vi "Test_State_Block_Chain.vi"() -> ()   [LabVIEW 2021]
uses:
  C:/Program Files (x86)/Hyper State Machine Framework/SSW_Hyper_State_Machine.lvlibp/State_Machine_Class/Main_State_Machine/Hyper_State_Machine.lvclass
  C:/Program Files (x86)/Hyper State Machine Framework/SSW_Hyper_State_Machine.lvlibp/State_Interface/State_Interface.lvclass
  Motion_Panel_State_Machine/Motion_Panel_State_Machine.lvclass
  C:/Program Files (x86)/Hyper State Machine Framework/SSW_Panel_Adaptive.lvlibp/Panel_Adaptive/Panel_Adaptive.lvclass
  C:/Program Files (x86)/Hyper State Machine Framework/SSW_Panel_Adaptive.lvlibp/Panel_Interface/Panel_Interface.lvclass
  DIO_Panel_State_Machine/DIO_Panel_State_Machine.lvclass
  Class 1/Panel1.lvclass
  Class 3/Panel3.lvclass
  Class 2/Panel2.lvclass
  C:/Program Files (x86)/Hyper State Machine Framework/SSW_Hyper_State_Machine.lvlibp/State_Machine_Class/State_Machine_Module.llb/State Machine.ctl
  C:/Program Files (x86)/Hyper State Machine Framework/SSW_Hyper_State_Machine.lvlibp/State_Machine_Class/State_Machine_Module.llb/State Machine[].ctl
  C:/Program Files (x86)/Hyper State Machine Framework/SSW_Hyper_State_Machine.lvlibp/State_Machine_Class/State_Machine_Module.llb/Time_Out.ctl
  C:/Program Files (x86)/Hyper State Machine Framework/SSW_Hyper_State_Machine.lvlibp/State_Machine_Class/State_Machine_Module.llb/Lock_Unlock.ctl
  C:/Program Files (x86)/Hyper State Machine Framework/SSW_Hyper_State_Machine.lvlibp
panel:
  out "Parent_State":refnum<class "Hyper_State_Machine.lvclass">
  out "HPSMO4-20":refnum<class "Panel_Adaptive.lvclass">[](array[class])
  out "HPSMO2":refnum<class "Panel_Adaptive.lvclass">
  out "HSMO4-20":refnum<class "Hyper_State_Machine.lvclass">[](array[class])
  out "HSMO3":refnum<class "Hyper_State_Machine.lvclass">
  out "HPSMO3":refnum<class "DIO_Panel_State_Machine.lvclass">
  out "HSMO2":refnum<class "Hyper_State_Machine.lvclass">
  out "HSMO1":refnum<class "Hyper_State_Machine.lvclass">
  out "HPSMO1":refnum<class "Motion_Panel_State_Machine.lvclass">
  in  "Reset_State":bool
  in  "Reset_All":bool
  in  "Change_VI_All":bool
  in  "Panel Index":i32=1 min=1 max=20
  in  "Implementation":u16(ring)
  in  "Change_VI":bool
  out "Main_Active":bool
  in  "Main_Interval(s)":dbl=0.025 format="%.0p"
  in  "Option Button":bool=TRUE
  in  "Time Target (s)":dbl=30.0 format="%#_13g"
  in  "lock All":bool
  in  "Unlock":bool
  out "All_Values":variant[][](array[variant])
  out "error out":errorcluster
  in  "Exit":bool
  in  "Tab Control":T1(tab)
  in  "Panel Mode 4":bool
  in  "Panel Mode 3":bool
  in  "Panel Mode 2":bool
  in  "Panel Mode 1":bool
  in  "Swap3-4":bool
  in  "Swap1-4":bool
  in  "Swap2-3":bool
  in  "Swap1-2":bool
  out "Active 3":bool
  out "Active 2":bool
  out "Timing 3":dbl
  out "Timing 2":dbl
  out "Active 1":bool
  out "Timing 1":dbl
  out "Timing 20":dbl
  out "Active 20":bool
  out "Get_Current State_Sub Panel_1":string
  out "Sub Panel_1(HSMO_ID)":u32 format="%08x"
  out "HSMO1 Running":bool
  in  "Request_Release(Index)":bool
  out "Block_Chain_Lock":bool
  out "Current_Parent_State":string
  out "Parent_State_ID":u32 format="%08x"
  out "Received State Message":string
  out "Child_State#":u32
  out "Child_State_ID":u32[](array[numeric]) format="%.0x"
  in  "Panel_Index":u32 max=3 step=1
  # "Local"
  # "Panel Method"
  # "State Method"
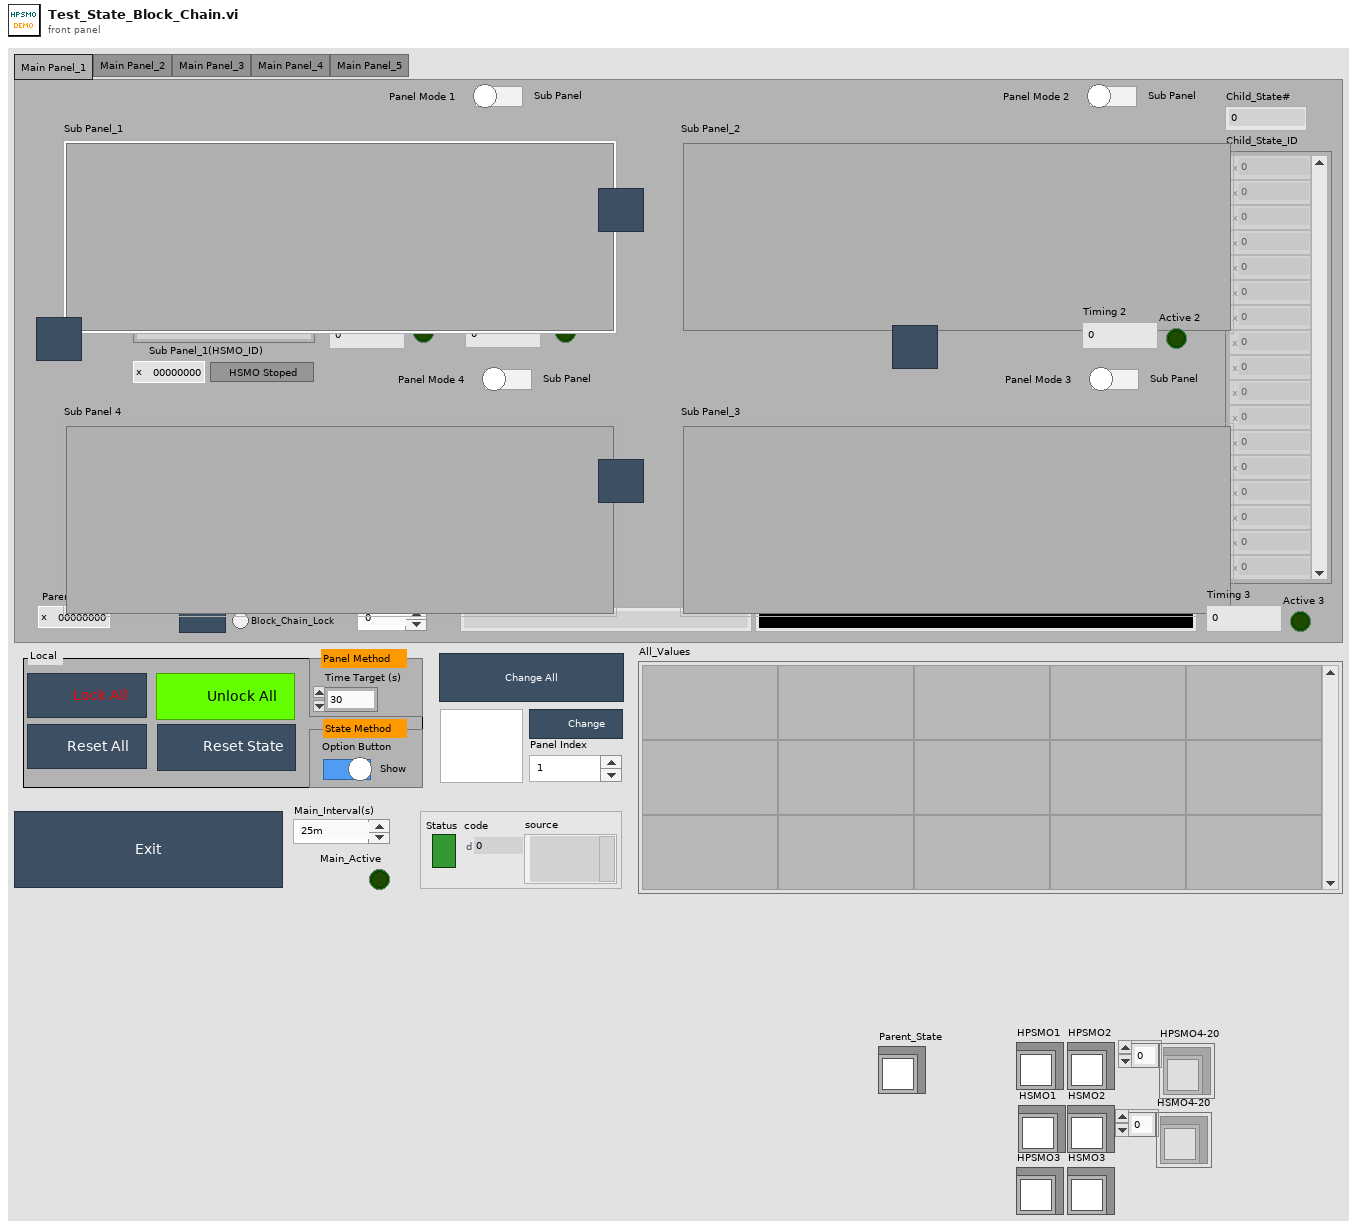
[diagram p1: front panel]
types:
  T1 = enum32{"Main Panel_1", "Main Panel_2", "Main Panel_3", "Main Panel_4", "Main Panel_5"}
  T2 = typedef "SSW_Hyper_State_Machine.lvlibp/State Machine.ctl" = cluster{"Command":string, "Data":variant}
  T3 = typedef "SSW_Hyper_State_Machine.lvlibp/Lock_Unlock.ctl" = cluster{"Action_Mode (Get)":enum16{"Set", "Get"}, "Action_Set (False)":bool, "State_In (Wait)":string}
  T4 = typedef "SSW_Hyper_State_Machine.lvlibp/State Machine[].ctl" = cluster{"Command":string, "Data":variant}[]
  T5 = typedef "SSW_Hyper_State_Machine.lvlibp/Time_Out.ctl" = cluster{"Enable(True)":bool, "Time Out_State Name":string, "Time Target (1s)":dbl, "Time Out_Reply Message_State":string}
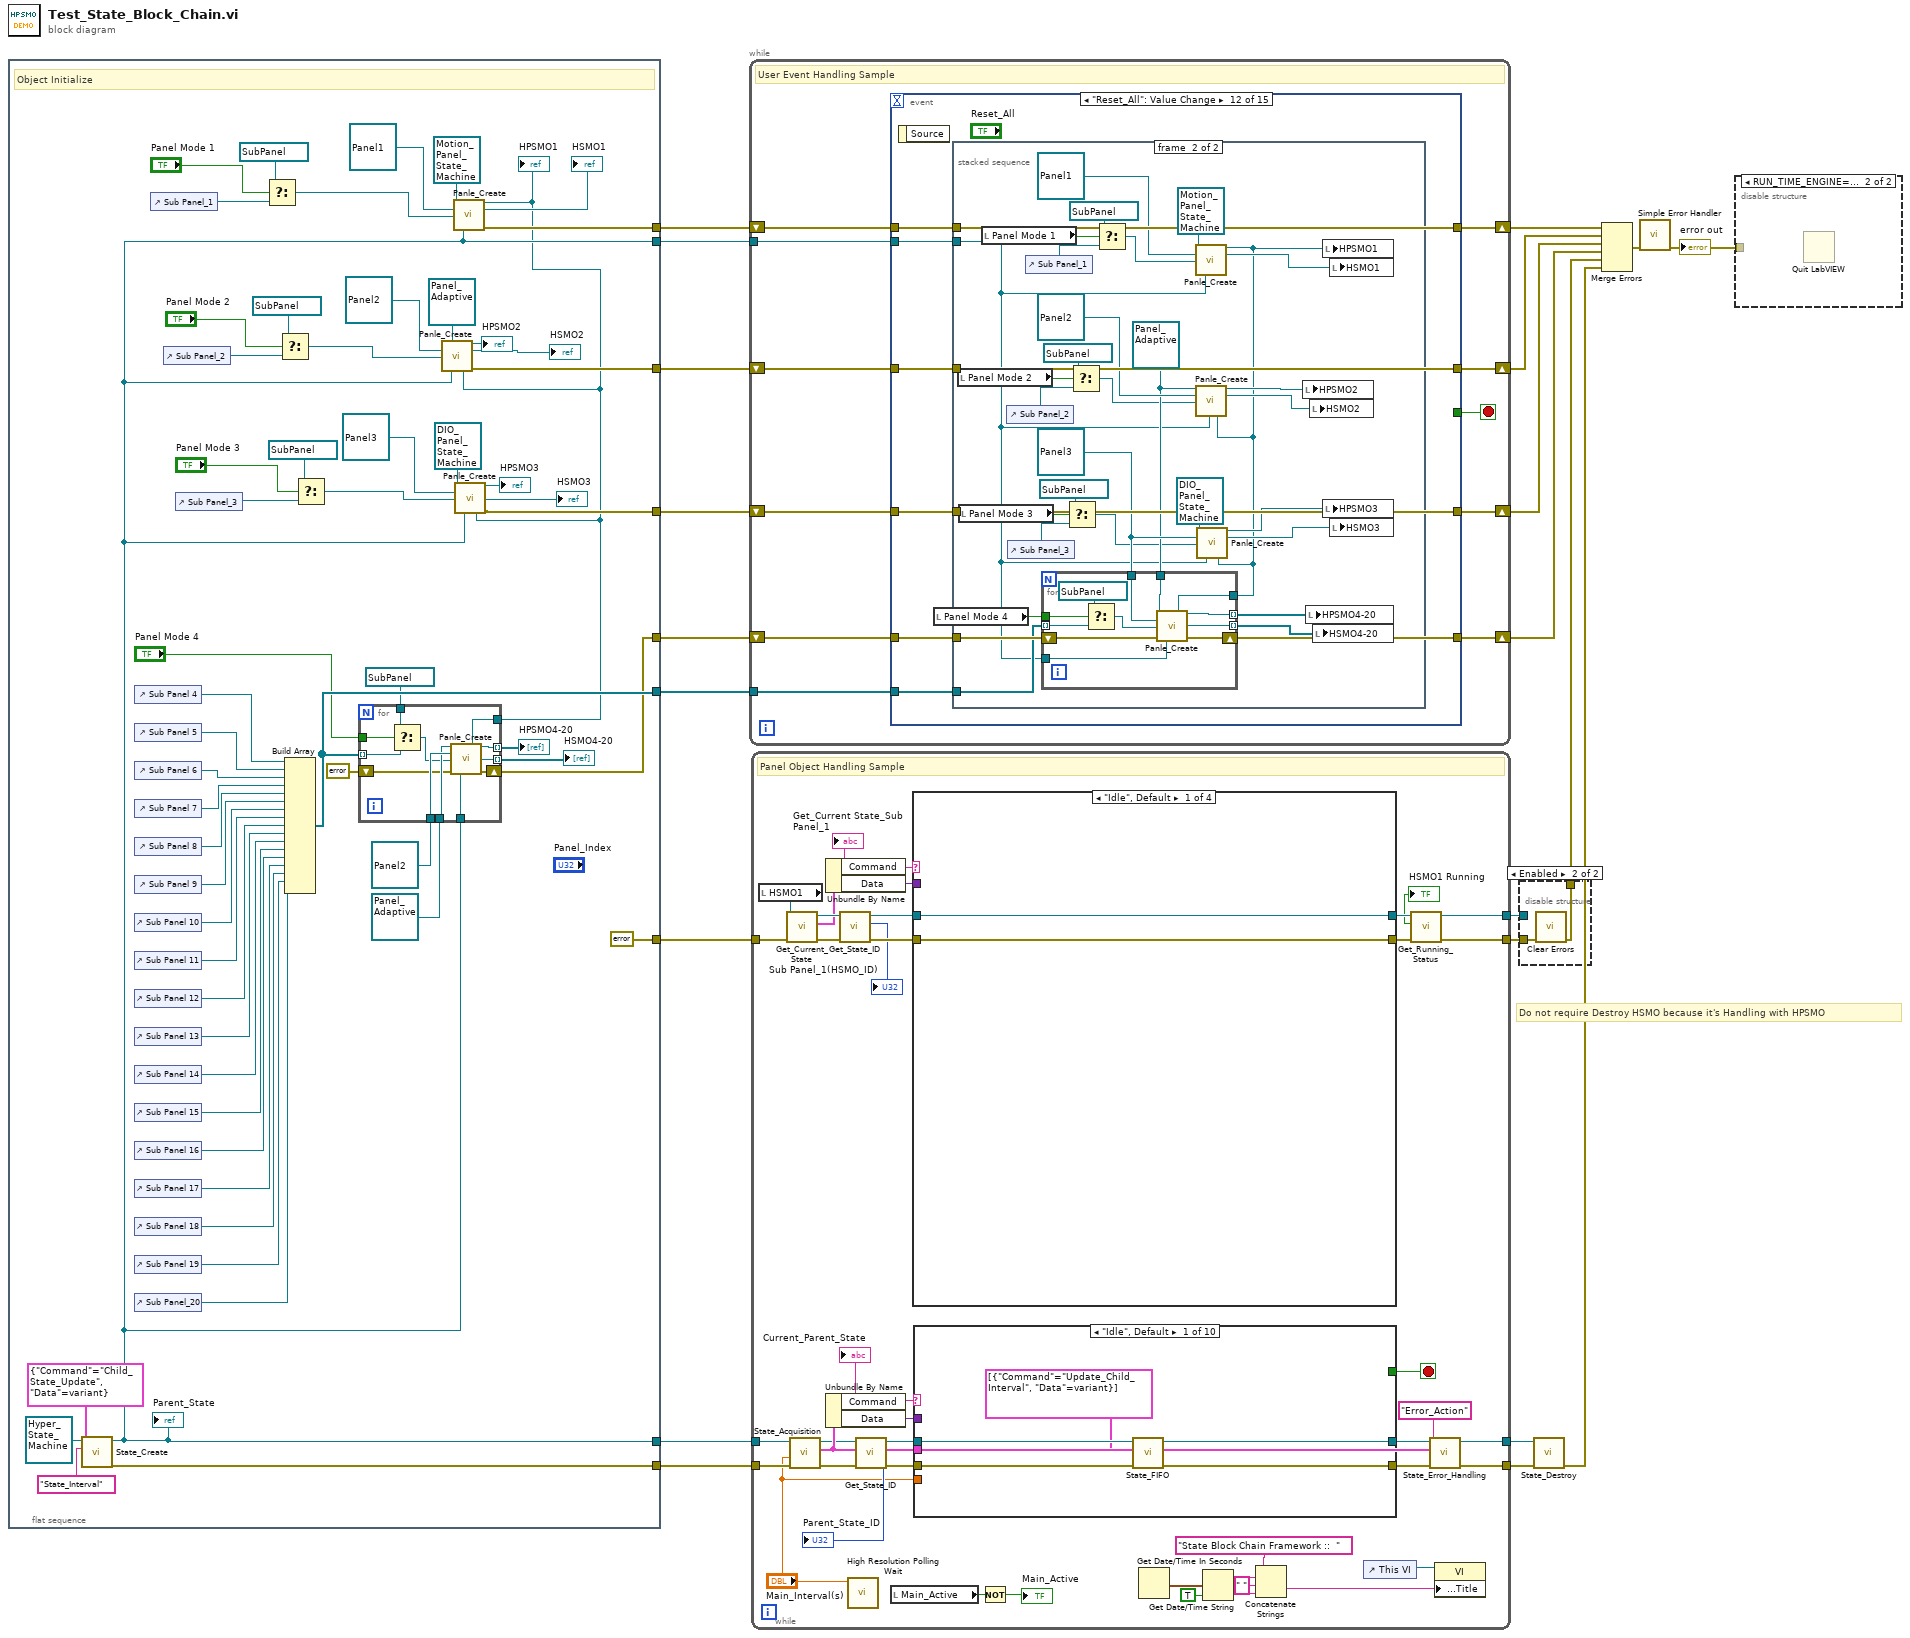
[diagram p0: block diagram]
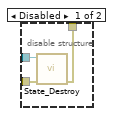
[diagram p2: hidden frame]
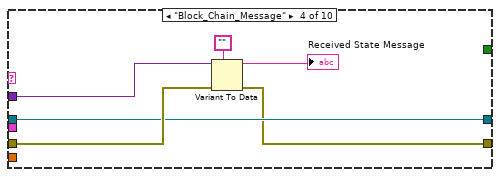
[diagram p6: hidden frame]
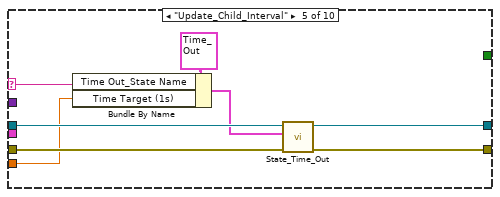
[diagram p7: hidden frame]
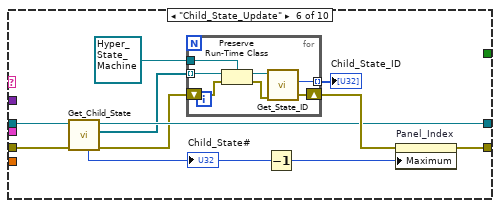
[diagram p8: hidden frame]
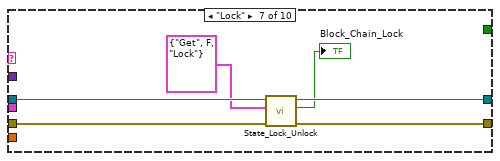
[diagram p9: hidden frame]
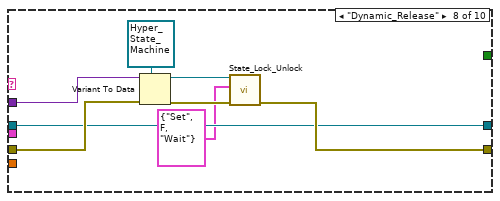
[diagram p10: hidden frame]
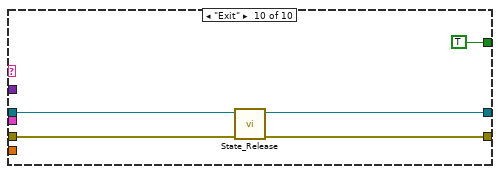
[diagram p12: hidden frame]
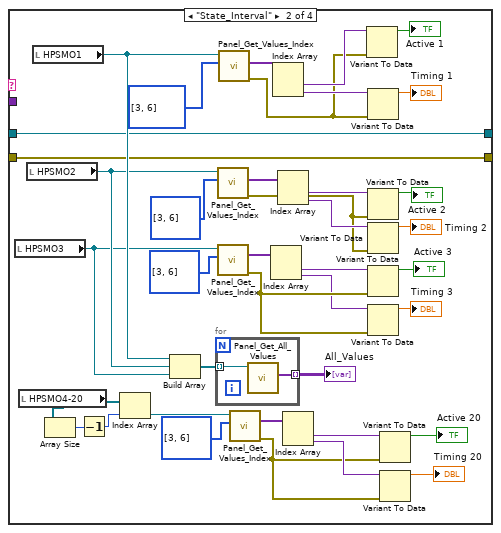
[diagram p13: hidden frame]
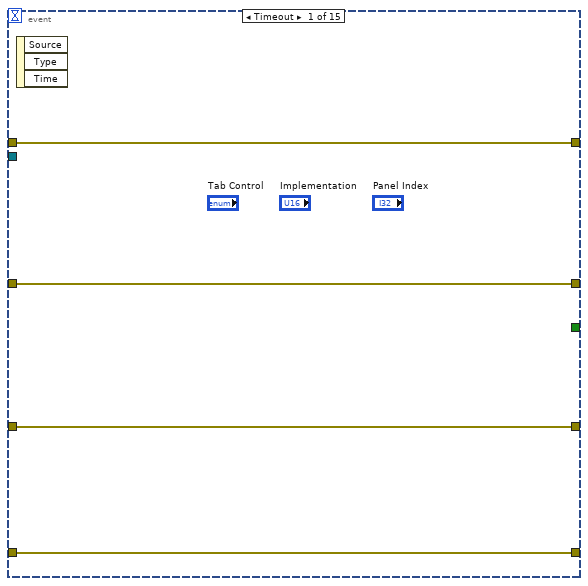
[diagram p16: hidden frame]
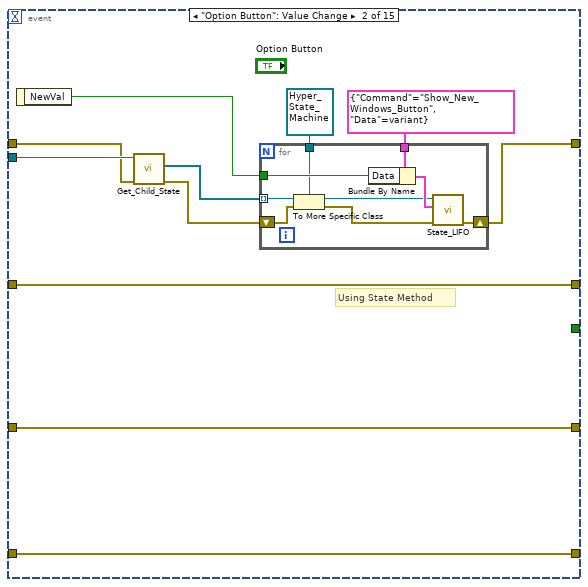
[diagram p17: hidden frame]
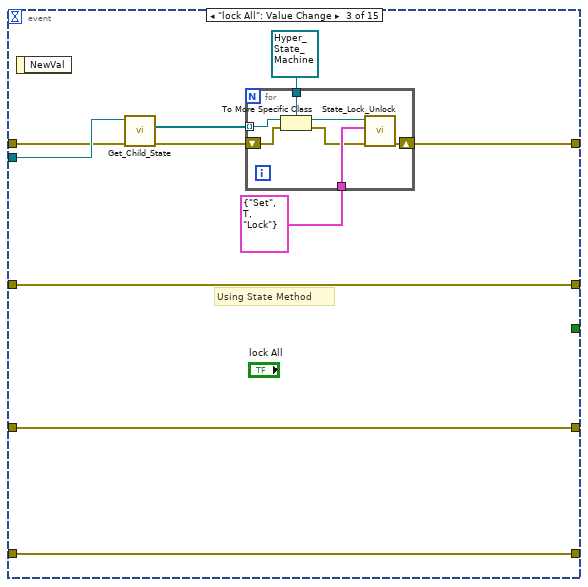
[diagram p18: hidden frame]
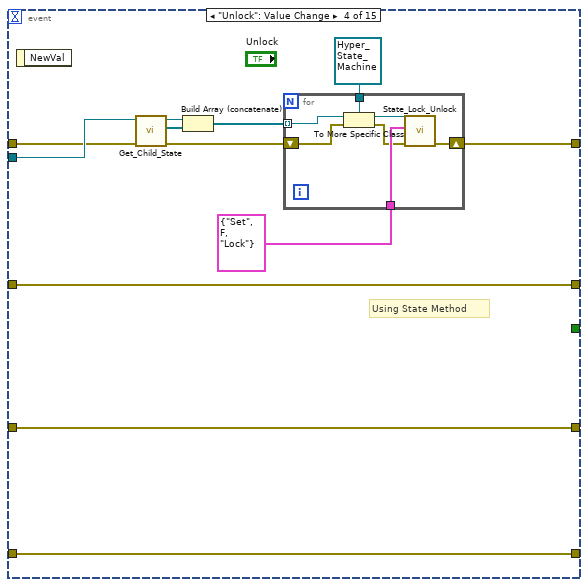
[diagram p19: hidden frame]
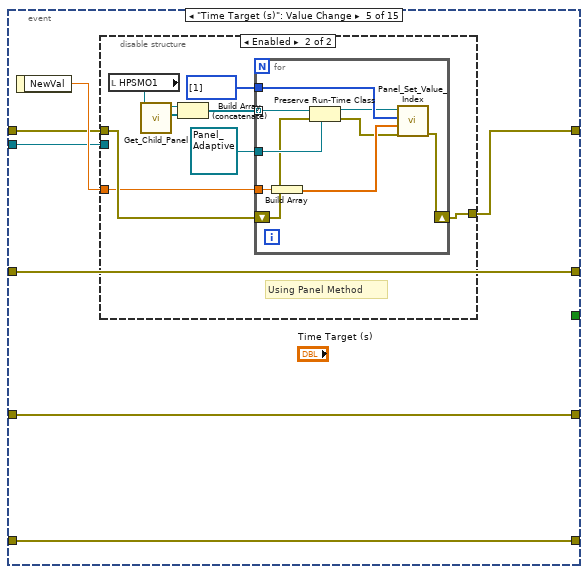
[diagram p20: hidden frame]
diagram:
  # "Do not require Destroy HSMO because it's Handling with HPSMO"
  n1 = flat-sequence {
    tunnel: [w55] -> w21
    tunnel: [w53] -> w10
    tunnel: [w52] -> w7
    tunnel: [w51] -> w8
    tunnel: [w46] -> w9
    tunnel: [errorcluster {"status"=FALSE, "code"=0, "source"=""} ("error in (no error)")] -> w14
    tunnel: [w37] -> w13
    tunnel: [w39] -> w12
    tunnel: [w37] -> w11
    frame #0 {
      # "Object Initialize"
      n2 = call-dynamic "State_Create.vi"("Init_State(Option)"=T2 {"Command"="Child_State_Update", "Data"=variant}, "State_Interval_Name"="State_Interval", "State_Machine_Class in"=refnum<class "Hyper_State_Machine.lvclass"> refnum) -> ("error out"=w39:errorcluster, "State_Machine_Class out"=w37:refnum<class "Hyper_State_Machine.lvclass">)  [unwired: 6 in, 1 out]
      "Parent_State" <- w37
      n3 = control-ref of="Sub Panel 4"() -> (w75:refnum<vi>)
      n4 = control-ref of="Sub Panel 5"() -> (w74:refnum<vi>)
      n5 = control-ref of="Sub Panel 6"() -> (w73:refnum<vi>)
      n6 = control-ref of="Sub Panel 7"() -> (w72:refnum<vi>)
      n7 = control-ref of="Sub Panel 8"() -> (w71:refnum<vi>)
      n8 = control-ref of="Sub Panel 9"() -> (w70:refnum<vi>)
      n9 = control-ref of="Sub Panel 10"() -> (w69:refnum<vi>)
      n10 = control-ref of="Sub Panel 11"() -> (w68:refnum<vi>)
      n11 = control-ref of="Sub Panel 12"() -> (w67:refnum<vi>)
      n12 = control-ref of="Sub Panel 13"() -> (w66:refnum<vi>)
      n13 = control-ref of="Sub Panel 14"() -> (w65:refnum<vi>)
      n14 = control-ref of="Sub Panel 15"() -> (w64:refnum<vi>)
      n15 = control-ref of="Sub Panel 16"() -> (w63:refnum<vi>)
      n16 = control-ref of="Sub Panel 17"() -> (w62:refnum<vi>)
      n17 = control-ref of="Sub Panel 18"() -> (w61:refnum<vi>)
      n18 = control-ref of="Sub Panel 19"() -> (w60:refnum<vi>)
      n19 = control-ref of="Sub Panel_20"() -> (w58:refnum<vi>)
      n20 = control-ref of="Sub Panel_1"() -> (w35:refnum<vi>)
      n21 = control-ref of="Sub Panel_2"() -> (w30:refnum<vi>)
      n22 = control-ref of="Sub Panel_3"() -> (w26:refnum<vi>)
      n23 = Select(t=refnum<vi> refnum, s="Panel Mode 1", f=w35) -> (s? t:f=w34:refnum<vi>)
      n24 = Select(t=refnum<vi> refnum, s="Panel Mode 2", f=w30) -> (s? t:f=w28:refnum<vi>)
      n25 = Build Array(w75, w74, w73, w72, w71, w70, w69, w68, w67, w66, w65, w64, w63, w62, w61, w60, w58) -> (w55:refnum<vi>[])
      n26 = Select(t=refnum<vi> refnum, s="Panel Mode 3", f=w26) -> (s? t:f=w25:refnum<vi>)
      n27 = call-dynamic "Panle_Create.vi"("Hyper_Panel_State_Machine in"=refnum<class "Motion_Panel_State_Machine.lvclass"> refnum ("Motion_Panel_State_Machine.lvclass"), "Panel_Source"=refnum<class "Panel1.lvclass"> refnum ("Class 1.lvclass"), "Panel_Ref"=w34, "Parent_State"=w37) -> ("Hyper_Panel_State_Machine out"=w22:refnum<class "Motion_Panel_State_Machine.lvclass">, "This_State"=→"HSMO1":refnum<class "Hyper_State_Machine.lvclass">, "error out"=w53:errorcluster)  [unwired: 9 in]
      "HPSMO1" <- w22
      n28 = for {
        shift-right: [w89] -> w52
        shift-left: errorcluster {"status"=FALSE, "code"=0, "source"=""} ("error out") -> [w90]
        tunnel: w55 -> [w84] mode=indexing
        tunnel: [w88] -> w59 mode=indexing
        tunnel: refnum<class "Panel2.lvclass"> refnum ("Class 2.lvclass") -> [w92]
        tunnel: refnum<class "Panel_Adaptive.lvclass"> refnum ("SSW_Panel_Adaptive.lvlibp:Panel_Adaptive.lvclass") -> [w91]
        tunnel: [w87] -> w44 mode=indexing
        tunnel: w37 -> [w86]
        tunnel: "Panel Mode 4" -> [w85]
        tunnel: refnum<vi> refnum ("t") -> [w83]
        tunnel: w22 -> [w81]
        n29 = Select(t=w83, s=w85, f=w84) -> (s? t:f=w82:refnum<vi>)
        n30 = call-dynamic "Panle_Create.vi"("Hyper_Panel_State_Machine in"=w91, "Panel_Source"=w92, "Panel_Ref"=w82, "error in (no error)"=w90, "Parent_State"=w86, "Parent_Panel"=w81) -> ("Hyper_Panel_State_Machine out"=w87:refnum<class "Panel_Adaptive.lvclass">, "This_State"=w88:refnum<class "Hyper_State_Machine.lvclass">, "error out"=w89:errorcluster)  [unwired: 7 in]
      }
      "HSMO4-20" <- w59
      "HPSMO4-20" <- w44
      n31 = call-dynamic "Panle_Create.vi"("Hyper_Panel_State_Machine in"=refnum<class "Panel_Adaptive.lvclass"> refnum ("SSW_Panel_Adaptive.lvlibp:Panel_Adaptive.lvclass"), "Panel_Source"=refnum<class "Panel2.lvclass"> refnum ("Class 2.lvclass"), "Panel_Ref"=w28, "Parent_State"=w37, "Parent_Panel"=w22) -> ("Hyper_Panel_State_Machine out"=→"HPSMO2":refnum<class "Panel_Adaptive.lvclass">, "This_State"=→"HSMO2":refnum<class "Hyper_State_Machine.lvclass">, "error out"=w46:errorcluster)  [unwired: 8 in]
      n32 = call-dynamic "Panle_Create.vi"("Hyper_Panel_State_Machine in"=refnum<class "DIO_Panel_State_Machine.lvclass"> refnum ("DIO_Panel_State_Machine.lvclass"), "Panel_Source"=refnum<class "Panel3.lvclass"> refnum ("Class 3.lvclass"), "Panel_Ref"=w25, "Parent_State"=w37, "Parent_Panel"=w22) -> ("Hyper_Panel_State_Machine out"=→"HPSMO3":refnum<class "DIO_Panel_State_Machine.lvclass">, "This_State"=→"HSMO3":refnum<class "Hyper_State_Machine.lvclass">, "error out"=w51:errorcluster)  [unwired: 8 in]
    }
  }
  n33 = while {
    tunnel: w21 -> [w102]
    tunnel: w11 -> [w101]
    shift-right: [w93] -> w3
    shift-left: w10 -> [w100]
    shift-right: [w94] -> w4
    shift-left: w9 -> [w99]
    shift-right: [w95] -> w5
    shift-left: w8 -> [w98]
    shift-right: [w96] -> w6
    shift-left: w7 -> [w97]
    stop <- w103 stop-if-true
    # "User Event Handling Sample"
    n34 = event shown="[11] \"Reset_All\": Value Change" {
      selector: _ -> [_ _ _ _ _ _ _ _ _ _ _ _ _ _ _]
      dyn-events: _ -> [_ _ _ _ _ _ _ _ _ _ _ _ _ _ _]
      timeout: _ -> [_ _ _ _ _ _ _ _ _ _ _ _ _ _ _]
      tunnel: [_ _ _ _ _ _ _ _ _ _ _ _ _ _ w384] -> w103
      tunnel: w100 -> [w105 w110 w130 w148 w168 w213 _ w252 w257 w273 w281 w290 w348 w376 w392]
      tunnel: [_ w118 w137 w156 w170 w219 w232 w251 w257 w270 w281 w290 w351 w380 w390] -> w93
      tunnel: w99 -> [w106 w115 w135 w154 w165 _ _ w247 w262 w268 w282 w289 w355 _ w387]
      tunnel: [w105 _ _ _ _ _ _ _ _ _ _ _ _ _ _] -> _
      tunnel: [w106 w115 w135 w154 w165 w219 w232 w250 w260 w268 w282 w289 w355 _ w389] -> w94
      tunnel: [w107 w114 w134 w153 w166 w219 w232 w249 w259 w269 w280 w288 w354 _ w388] -> w95
      tunnel: w97 -> [w104 w113 w133 w152 w167 _ _ w248 w258 w272 w284 w287 w353 _ w386]
      tunnel: [w104 w113 w133 w152 w167 w219 w232 w248 w258 w271 w283 w287 w353 _ w385] -> w96
      tunnel: w98 -> [w107 w114 w134 w153 w166 _ _ w249 w261 w269 w279 w288 w354 _ w391]
      tunnel: w102 -> [_ _ _ _ _ _ _ _ _ _ _ w286 _ _ _]
      tunnel: w101 -> [_ w111 w131 w149 w164 _ _ _ _ _ _ w285 w349 w377 w382]
      event Timeout {
        n35 = event-data() -> ()  [unwired: 1 in, 3 out]
      }
      event "Option Button": Value Change {
        # "Using State Method"
        n36 = event-data() -> ("NewVal"=w117:bool)  [unwired: 1 in]
        n37 = call-dynamic "Get_Child_State.vi"("error in (no error)"=w110, "Hyper_State_Machine in"=w111) -> ("error out"=w108:errorcluster, "Child_State"=w109:refnum<class "State_Interface.lvclass">[])  [unwired: 5 in, 3 out]
        n38 = for {
          tunnel: w117 -> [w126]
          tunnel: w109 -> [w123] mode=indexing
          shift-right: [w127] -> w118
          shift-left: w108 -> [w120]
          tunnel: T2 {"Command"="Show_New_Windows_Button", "Data"=variant} ("State Machine") -> [w124]
          tunnel: refnum<class "Hyper_State_Machine.lvclass"> refnum ("HSMO1") -> [w122]
          n39 = To More Specific Class(target class=w122, reference=w123, error in=w120) -> (specific class reference=w121:refnum<class "Hyper_State_Machine.lvclass">, error out=w119:errorcluster)
          n40 = Bundle By Name(cluster=w124, "Data"=w126) -> (w125:T2)
          n41 = call-dynamic "State_LIFO.vi"("error in (no error)"=w119, "State Machine"=w125, "State_Machine_Class in"=w121) -> ("error out"=w127:errorcluster)  [unwired: 7 in, 1 out]
        }
      }
      event "lock All": Value Change {
        # "Using State Method"
        n42 = event-data() -> ()  [unwired: 1 in, 1 out]
        n43 = call-dynamic "Get_Child_State.vi"("error in (no error)"=w130, "Hyper_State_Machine in"=w131) -> ("error out"=w128:errorcluster, "Child_State"=w129:refnum<class "State_Interface.lvclass">[])  [unwired: 5 in, 3 out]
        n44 = for {
          shift-right: [w144] -> w137
          shift-left: w128 -> [w139]
          tunnel: T3 {"Action_Mode (Get)"=enum."Set", "Action_Set (False)"=TRUE, "State_In (Wait)"="Lock"} ("Parameter") -> [w143]
          tunnel: refnum<class "Hyper_State_Machine.lvclass"> refnum ("HSMO1") -> [w142]
          tunnel: w129 -> [w140] mode=indexing
          n45 = To More Specific Class(target class=w142, reference=w140, error in=w139) -> (specific class reference=w141:refnum<class "Hyper_State_Machine.lvclass">, error out=w138:errorcluster)
          n46 = call-dynamic "State_Lock_Unlock.vi"("error in (no error)"=w138, "Parameter"=w143, "State_Machine_Class in"=w141) -> ("error out"=w144:errorcluster)  [unwired: 6 in, 2 out]
        }
      }
      event "Unlock": Value Change {
        # "Using State Method"
        n47 = event-data() -> ()  [unwired: 1 in, 1 out]
        n48 = call-dynamic "Get_Child_State.vi"("error in (no error)"=w148, "Hyper_State_Machine in"=w149) -> ("error out"=w147:errorcluster, "Child_State"=w145:refnum<class "State_Interface.lvclass">[], "Hyper_State_Machine out"=w146:refnum<class "Hyper_State_Machine.lvclass">)  [unwired: 5 in, 2 out]
        n49 = Build Array (concatenate)(w146, w145) -> (w150:refnum<class "State_Interface.lvclass">[])
        n50 = for {
          shift-right: [w163] -> w156
          shift-left: w147 -> [w158]
          tunnel: T3 {"Action_Mode (Get)"=enum."Set", "Action_Set (False)"=FALSE, "State_In (Wait)"="Lock"} ("Parameter") -> [w162]
          tunnel: refnum<class "Hyper_State_Machine.lvclass"> refnum ("HSMO1") -> [w161]
          tunnel: w150 -> [w157] mode=indexing
          n51 = To More Specific Class(target class=w161, reference=w157, error in=w158) -> (specific class reference=w160:refnum<class "Hyper_State_Machine.lvclass">, error out=w159:errorcluster)
          n52 = call-dynamic "State_Lock_Unlock.vi"("error in (no error)"=w159, "Parameter"=w162, "State_Machine_Class in"=w160) -> ("error out"=w163:errorcluster)  [unwired: 6 in, 2 out]
        }
      }
      event "Time Target (s)": Value Change {
        n53 = event-data() -> ("NewVal"=w169:dbl)  [unwired: 1 in]
        n54 = disable-structure shown="Enabled" {
          disable-tunnel: [w177 w194] -> w170
          disable-tunnel: w169 -> [w178 w195]
          disable-tunnel: w168 -> [w173 w196]
          disable-tunnel: w164 -> [w174 _]
          frame Disabled {
            # "Using State Method"
            n55 = call-dynamic "Get_Child_State.vi"("error in (no error)"=w173, "Hyper_State_Machine in"=w174) -> ("error out"=w172:errorcluster, "Child_State"=w171:refnum<class "State_Interface.lvclass">[])  [unwired: 5 in, 3 out]
            n56 = for {
              tunnel: w178 -> [w187]
              shift-right: [w186] -> w177
              shift-left: w172 -> [w180]
              tunnel: T2 {"Command"="Change_Time_Target", "Data"=variant} ("State Machine") -> [w184]
              tunnel: w171 -> [w183] mode=indexing
              tunnel: refnum<class "Hyper_State_Machine.lvclass"> refnum ("HSMO1") -> [w181]
              n57 = To More Specific Class(target class=w181, reference=w183, error in=w180) -> (specific class reference=w182:refnum<class "Hyper_State_Machine.lvclass">, error out=w179:errorcluster)
              n58 = Bundle By Name(cluster=w184, "Data"=w187) -> (w185:T2)
              n59 = call-dynamic "State_LIFO.vi"("error in (no error)"=w179, "State Machine"=w185, "State_Machine_Class in"=w182) -> ("error out"=w186:errorcluster)  [unwired: 7 in, 1 out]
            }
          }
          frame Enabled {
            # "Using Panel Method"
            n60 = local read "HPSMO1"() -> (w188:refnum<class "Motion_Panel_State_Machine.lvclass">)
            n61 = call-dynamic "Get_Child_Panel.vi"("Motion_Panel_State_Machine in"=w188) -> ("Child_Panel"=w192:refnum<class "Panel_Interface.lvclass">[], "Motion_Panel_State_Machine out"=w191:refnum<class "Motion_Panel_State_Machine.lvclass">)  [unwired: 6 in, 3 out]
            n62 = Build Array (concatenate)(w191, w192) -> (w190:refnum<class "Panel_Interface.lvclass">[])
            n63 = for {
              tunnel: w190 -> [w201] mode=indexing
              tunnel: w195 -> [w205]
              shift-right: [w202] -> w194
              shift-left: w196 -> [w199]
              tunnel: i32[] [1] ("Control_Indexes(Tabbing Order)") -> [w204]
              tunnel: refnum<class "Panel_Adaptive.lvclass"> refnum ("SSW_Panel_Adaptive.lvlibp:Panel_Adaptive.lvclass") -> [w200]
              n64 = Build Array(w205) -> (w203:dbl[])
              n65 = Preserve Run-Time Class(object in=w201, error in=w199, 2:w200) -> (object out=w198:refnum<class "Panel_Adaptive.lvclass">, error out=w197:errorcluster)
              n66 = call-dynamic "Panel_Set_Value_Index.vi"("error in (no error)"=w197, "Data_Values"=w203, "Control_Indexes(Tabbing Order)"=w204, "Hyper_Panel_State_Machine in"=w198) -> ("error out"=w202:errorcluster)  [unwired: 6 in, 1 out]
            }
          }
        }
      }
      event "Change_VI": Value Change {
        n67 = event-data() -> ()  [unwired: 1 in, 1 out]
        n68 = local read "Implementation"() -> (w217:u16)
        n69 = local read "HPSMO1"() -> (w206:refnum<class "Motion_Panel_State_Machine.lvclass">)
        n70 = local read "Panel Index"() -> (w218:i32)
        n71 = call-dynamic "Get_Child_Panel.vi"("error in (no error)"=w213, "Motion_Panel_State_Machine in"=w206) -> ("error out"=w208:errorcluster, "Child_Panel"=w215:refnum<class "Panel_Interface.lvclass">[], "Motion_Panel_State_Machine out"=w214:refnum<class "Motion_Panel_State_Machine.lvclass">)  [unwired: 5 in, 2 out]
        n72 = Build Array (concatenate)(w214, w215) -> (w212:refnum<class "Panel_Interface.lvclass">[])
        n73 = case shown="1" w217 {
          tunnel: [refnum<class "Panel1.lvclass"> refnum ("Class 1.lvclass") refnum<class "Panel2.lvclass"> refnum ("Class 2.lvclass") refnum<class "Panel3.lvclass"> refnum ("Class 3.lvclass")] -> w216
          frame 0, Default {
          }
          frame 1 {
          }
          frame 2 {
          }
        }
        n74 = Decrement(x=w218) -> (x-1=w220:i32)
        n75 = Index Array(array=w212, index=w220) -> (element=w211:refnum<class "Panel_Interface.lvclass">)
        n76 = Preserve Run-Time Class(object in=w211, error in=w208, 2:refnum<class "Panel_Adaptive.lvclass"> refnum ("SSW_Panel_Adaptive.lvlibp:Panel_Adaptive.lvclass")) -> (object out=w210:refnum<class "Panel_Adaptive.lvclass">, error out=w207:errorcluster)
        n77 = call-dynamic "Panel_Change.vi"("error in (no error)"=w207, "Panel_Source"=w216, "Hyper_Panel_State_Machine in"=w210) -> ("error out"=w219:errorcluster)  [unwired: 7 in, 1 out]
      }
      event "Change_VI_All": Value Change {
        n78 = event-data() -> ()  [unwired: 1 in, 1 out]
        n79 = local read "HPSMO1"() -> (w224:refnum<class "Motion_Panel_State_Machine.lvclass">)
        n80 = local read "Implementation"() -> (w231:u16)
        n81 = call-dynamic "Get_Child_Panel.vi"("Motion_Panel_State_Machine in"=w224) -> ("Child_Panel"=w228:refnum<class "Panel_Interface.lvclass">[], "Motion_Panel_State_Machine out"=w227:refnum<class "Motion_Panel_State_Machine.lvclass">)  [unwired: 6 in, 3 out]
        n82 = Build Array (concatenate)(w227, w228) -> (w226:refnum<class "Panel_Interface.lvclass">[])
        n83 = case shown="0, Default" w231 {
          tunnel: [refnum<class "Panel1.lvclass"> refnum ("Class 1.lvclass") refnum<class "Panel2.lvclass"> refnum ("Class 2.lvclass") refnum<class "Panel3.lvclass"> refnum ("Class 3.lvclass")] -> w230
          frame 0, Default {
          }
          frame 1 {
          }
          frame 2 {
          }
        }
        n84 = for {
          tunnel: w226 -> [w237] mode=indexing
          tunnel: w230 -> [w238]
          shift-right: [w239] -> w232
          shift-left: errorcluster {"status"=FALSE, "code"=0, "source"=""} ("error out") -> [w235]
          tunnel: refnum<class "Panel_Adaptive.lvclass"> refnum ("SSW_Panel_Adaptive.lvlibp:Panel_Adaptive.lvclass") -> [w236]
          n85 = Preserve Run-Time Class(object in=w237, error in=w235, 2:w236) -> (object out=w234:refnum<class "Panel_Adaptive.lvclass">, error out=w233:errorcluster)
          n86 = call-dynamic "Panel_Change.vi"("error in (no error)"=w233, "Panel_Source"=w238, "Hyper_Panel_State_Machine in"=w234) -> ("error out"=w239:errorcluster)  [unwired: 7 in, 1 out]
        }
      }
      event "Swap1-2": Value Change {
        n87 = event-data() -> ()  [unwired: 1 in, 1 out]
        n88 = local read "HPSMO2"() -> (w244:refnum<class "Panel_Adaptive.lvclass">)
        n89 = local read "HPSMO1"() -> (w243:refnum<class "Motion_Panel_State_Machine.lvclass">)
        n90 = call-dynamic "Panel_Change.vi"("error in (no error)"=w252, "Interface_VI"=refnum<class "Panel2.lvclass"> refnum ("Class 2.lvclass"), "Hyper_Panel_State_Machine in"=w243) -> ("error out"=w251:errorcluster)  [unwired: 7 in, 1 out]
        n91 = call-dynamic "Panel_Change.vi"("error in (no error)"=w247, "Panel_Source"=refnum<class "Panel1.lvclass"> refnum ("Class 1.lvclass"), "Hyper_Panel_State_Machine in"=w244) -> ("error out"=w250:errorcluster)  [unwired: 7 in, 1 out]
      }
      event "Swap2-3": Value Change {
        n92 = event-data() -> ()  [unwired: 1 in, 1 out]
        n93 = local read "HPSMO1"() -> (w253:refnum<class "Motion_Panel_State_Machine.lvclass">)
        n94 = local read "HPSMO3"() -> (w254:refnum<class "DIO_Panel_State_Machine.lvclass">)
        n95 = call-dynamic "Panel_Change.vi"("error in (no error)"=w262, "Interface_VI"=refnum<class "Panel3.lvclass"> refnum ("Class 3.lvclass"), "Hyper_Panel_State_Machine in"=w253) -> ("error out"=w260:errorcluster)  [unwired: 7 in, 1 out]
        n96 = call-dynamic "Panel_Change.vi"("error in (no error)"=w261, "Interface_VI"=refnum<class "Panel2.lvclass"> refnum ("Class 2.lvclass"), "Hyper_Panel_State_Machine in"=w254) -> ("error out"=w259:errorcluster)  [unwired: 7 in, 1 out]
      }
      event "Swap1-4": Value Change {
        n97 = event-data() -> ()  [unwired: 1 in, 1 out]
        n98 = local read "HPSMO4-20"() -> (w265:refnum<class "Panel_Adaptive.lvclass">[])
        n99 = Index Array(array=w265) -> (element=w264:refnum<class "Panel_Adaptive.lvclass">)  [unwired: 1 in]
        n100 = local read "HPSMO1"() -> (w263:refnum<class "Motion_Panel_State_Machine.lvclass">)
        n101 = call-dynamic "Panel_Change.vi"("error in (no error)"=w273, "Interface_VI"=refnum<class "Panel3.lvclass"> refnum ("Class 3.lvclass"), "Hyper_Panel_State_Machine in"=w263) -> ("error out"=w270:errorcluster)  [unwired: 7 in, 1 out]
        n102 = call-dynamic "Panel_Change.vi"("error in (no error)"=w272, "Panel_Source"=refnum<class "Panel1.lvclass"> refnum ("Class 1.lvclass"), "Hyper_Panel_State_Machine in"=w264) -> ("error out"=w271:errorcluster)  [unwired: 7 in, 1 out]
      }
      event "Swap3-4": Value Change {
        n103 = event-data() -> ()  [unwired: 1 in, 1 out]
        n104 = local read "HPSMO4-20"() -> (w276:refnum<class "Panel_Adaptive.lvclass">[])
        n105 = Index Array(array=w276) -> (element=w275:refnum<class "Panel_Adaptive.lvclass">)  [unwired: 1 in]
        n106 = local read "HPSMO3"() -> (w274:refnum<class "DIO_Panel_State_Machine.lvclass">)
        n107 = call-dynamic "Panel_Change.vi"("error in (no error)"=w279, "Interface_VI"=refnum<class "Panel2.lvclass"> refnum ("Class 2.lvclass"), "Hyper_Panel_State_Machine in"=w274) -> ("error out"=w280:errorcluster)  [unwired: 7 in, 1 out]
        n108 = call-dynamic "Panel_Change.vi"("error in (no error)"=w284, "Panel_Source"=refnum<class "Panel3.lvclass"> refnum ("Class 3.lvclass"), "Hyper_Panel_State_Machine in"=w275) -> ("error out"=w283:errorcluster)  [unwired: 7 in, 1 out]
      }
      event "Reset_All": Value Change {
        n109 = event-data() -> ()  [unwired: 1 in, 1 out]
        n110 = stacked-sequence {
          tunnel: w290 -> [_ _]
          tunnel: w289 -> [_ _]
          tunnel: w288 -> [_ _]
          tunnel: w287 -> [w297 _]
          tunnel: w286 -> [_ w328]
          tunnel: w285 -> [_ w318]
          frame #0 {
            # "Remove Parent State with Last"
            n111 = local read "HPSMO1"() -> (w292:refnum<class "Motion_Panel_State_Machine.lvclass">)
            n112 = call-dynamic "Get_Child_Panel.vi"("error in (no error)"=w297, "Motion_Panel_State_Machine in"=w292) -> ("error out"=w296:errorcluster, "Child_Panel"=w294:refnum<class "Panel_Interface.lvclass">[], "Motion_Panel_State_Machine out"=w291:refnum<class "Motion_Panel_State_Machine.lvclass">)  [unwired: 5 in, 2 out]
            n113 = Build Array (concatenate)(w294, w291) -> (w295:refnum<class "Panel_Interface.lvclass">[])
            n114 = for {
              tunnel: w295 -> [w303] mode=indexing
              tunnel: refnum<class "Panel_Adaptive.lvclass"> refnum ("SSW_Panel_Adaptive.lvlibp:Panel_Adaptive.lvclass") -> [w301]
              tunnel: w296 -> [w302]
              tunnel: [w298] -> _
              n115 = Preserve Run-Time Class(object in=w303, error in=w302, 2:w301) -> (object out=w300:refnum<class "Panel_Adaptive.lvclass">, error out=w299:errorcluster)
              n116 = call-dynamic "Panel_Destroy.vi"("error in (no error)"=w299, "Hyper_Panel_State_Machine in"=w300) -> ("error out"=w298:errorcluster)  [unwired: 9 in]
            }
          }
          frame #1 {
            w319 = refnum<class "Panel_Adaptive.lvclass"> refnum ("SSW_Panel_Adaptive.lvlibp:Panel_Adaptive.lvclass")
            w329 = refnum<class "Panel3.lvclass"> refnum ("Class 3.lvclass")
            n117 = local read "Panel Mode 4"() -> (w308:bool)
            n118 = local read "Panel Mode 2"() -> (w306:bool)
            n119 = local read "Panel Mode 3"() -> (w307:bool)
            n120 = local read "Panel Mode 1"() -> (w305:bool)
            n121 = control-ref of="Sub Panel_2"() -> (w312:refnum<vi>)
            n122 = control-ref of="Sub Panel_3"() -> (w310:refnum<vi>)
            n123 = control-ref of="Sub Panel_1"() -> (w314:refnum<vi>)
            n124 = Select(t=refnum<vi> refnum, s=w307, f=w310) -> (s? t:f=w309:refnum<vi>)
            n125 = Select(t=refnum<vi> refnum, s=w306, f=w312) -> (s? t:f=w311:refnum<vi>)
            n126 = Select(t=refnum<vi> refnum, s=w305, f=w314) -> (s? t:f=w313:refnum<vi>)
            n127 = call-dynamic "Panle_Create.vi"("Hyper_Panel_State_Machine in"=refnum<class "Motion_Panel_State_Machine.lvclass"> refnum ("Motion_Panel_State_Machine.lvclass"), "Panel_Source"=refnum<class "Panel1.lvclass"> refnum ("Class 1.lvclass"), "Panel_Ref"=w313, "Parent_State"=w318) -> ("Hyper_Panel_State_Machine out"=w304:refnum<class "Motion_Panel_State_Machine.lvclass">, "This_State"=w326:refnum<class "Hyper_State_Machine.lvclass">)  [unwired: 9 in, 1 out]
            n128 = for {
              tunnel: w319 -> [w344]
              tunnel: [w343] -> w321 mode=indexing
              shift-right: [w341] -> _
              shift-left: _ -> [w342]
              tunnel: w328 -> [w335] mode=indexing
              tunnel: [w340] -> w320 mode=indexing
              tunnel: w329 -> [w339]
              tunnel: w318 -> [w338]
              tunnel: w308 -> [w334]
              tunnel: w304 -> [w333]
              n129 = Select(t=refnum<vi> refnum, s=w334, f=w335) -> (s? t:f=w336:refnum<vi>)
              n130 = call-dynamic "Panle_Create.vi"("Hyper_Panel_State_Machine in"=w344, "Panel_Source"=w339, "Panel_Ref"=w336, "error in (no error)"=w342, "Parent_State"=w338, "Parent_Panel"=w333) -> ("Hyper_Panel_State_Machine out"=w343:refnum<class "Panel_Adaptive.lvclass">, "This_State"=w340:refnum<class "Hyper_State_Machine.lvclass">, "error out"=w341:errorcluster)  [unwired: 7 in]
            }
            n131 = call-dynamic "Panle_Create.vi"("Hyper_Panel_State_Machine in"=w319, "Panel_Source"=refnum<class "Panel2.lvclass"> refnum ("Class 2.lvclass"), "Panel_Ref"=w311, "Parent_State"=w318, "Parent_Panel"=w304) -> ("Hyper_Panel_State_Machine out"=w325:refnum<class "Panel_Adaptive.lvclass">, "This_State"=w324:refnum<class "Hyper_State_Machine.lvclass">)  [unwired: 8 in, 1 out]
            n132 = call-dynamic "Panle_Create.vi"("Hyper_Panel_State_Machine in"=refnum<class "DIO_Panel_State_Machine.lvclass"> refnum ("DIO_Panel_State_Machine.lvclass"), "Panel_Source"=w329, "Panel_Ref"=w309, "Parent_State"=w318, "Parent_Panel"=w304) -> ("Hyper_Panel_State_Machine out"=w323:refnum<class "DIO_Panel_State_Machine.lvclass">, "This_State"=w322:refnum<class "Hyper_State_Machine.lvclass">)  [unwired: 8 in, 1 out]
            n133 = local write "HPSMO2"(w325) -> ()
            n134 = local write "HPSMO4-20"(w321) -> ()
            n135 = local write "HSMO2"(w324) -> ()
            n136 = local write "HSMO4-20"(w320) -> ()
            n137 = local write "HPSMO1"(w304) -> ()
            n138 = local write "HPSMO3"(w323) -> ()
            n139 = local write "HSMO1"(w326) -> ()
            n140 = local write "HSMO3"(w322) -> ()
          }
        }
      }
      event "Reset_State": Value Change {
        n141 = event-data() -> ()  [unwired: 1 in, 1 out]
        n142 = call-dynamic "Get_Child_State.vi"("error in (no error)"=w348, "Hyper_State_Machine in"=w349) -> ("error out"=w345:errorcluster, "Child_State"=w346:refnum<class "State_Interface.lvclass">[], "Hyper_State_Machine out"=w347:refnum<class "Hyper_State_Machine.lvclass">)  [unwired: 5 in, 2 out]
        n143 = Build Array (concatenate)(w347, w346) -> (w350:refnum<class "State_Interface.lvclass">[])
        n144 = for {
          tunnel: T2 {"Command"="State_Init", "Data"=variant} ("State Machine") -> [w363]
          tunnel: refnum<class "Hyper_State_Machine.lvclass"> refnum ("HSMO1") -> [w362]
          tunnel: w350 -> [w361] mode=indexing
          shift-right: [w357] -> w351
          shift-left: w345 -> [w358]
          n145 = To More Specific Class(target class=w362, reference=w361, error in=w358) -> (specific class reference=w360:refnum<class "Hyper_State_Machine.lvclass">, error out=w359:errorcluster)
          n146 = call-dynamic "State_Release.vi"("error in (no error)"=w359, "State_Machine_Class in"=w360) -> ("error out"=w364:errorcluster, "State_Machine_Class out"=w365:refnum<class "Hyper_State_Machine.lvclass">)  [unwired: 8 in]
          n147 = call-dynamic "State_LIFO.vi"("error in (no error)"=w364, "State Machine"=w363, "State_Machine_Class in"=w365) -> ("error out"=w357:errorcluster)  [unwired: 7 in, 1 out]
        }
      }
      event "Request_Release(Index)": Value Change {
        n148 = event-data() -> ()  [unwired: 1 in, 1 out]
        n149 = call-dynamic "State_Lock_Unlock.vi"("error in (no error)"=w376, "Parameter"=T3 {"Action_Mode (Get)"=enum."Set", "Action_Set (False)"=TRUE, "State_In (Wait)"="Lock"}, "State_Machine_Class in"=w377) -> ("error out"=w369:errorcluster, "State_Machine_Class out"=w370:refnum<class "Hyper_State_Machine.lvclass">)  [unwired: 6 in, 1 out]
        n150 = local read "Panel_Index"() -> (w372:u32)
        n151 = call-dynamic "Get_Child_State.vi"("error in (no error)"=w369, "Hyper_State_Machine in"=w370) -> ("error out"=w366:errorcluster, "Child_State"=w367:refnum<class "State_Interface.lvclass">[], "Hyper_State_Machine out"=w368:refnum<class "Hyper_State_Machine.lvclass">)  [unwired: 5 in, 2 out]
        n152 = Index Array(array=w367, index=w372) -> (element=w375:refnum<class "State_Interface.lvclass">)
        n153 = Bundle By Name(cluster=T2 {"Command"="Member_Release", "Data"=variant} ("State Machine"), "Data"=w368) -> (w378:T2)
        n154 = To More Specific Class(target class=refnum<class "Hyper_State_Machine.lvclass"> refnum ("State_Machine_Class out"), reference=w375, error in=w366) -> (specific class reference=w373:refnum<class "Hyper_State_Machine.lvclass">, error out=w371:errorcluster)
        n155 = call-dynamic "State_LIFO.vi"("error in (no error)"=w371, "State Machine"=w378, "State_Machine_Class in"=w373) -> ("error out"=w380:errorcluster)  [unwired: 7 in, 1 out]
      }
      event "Exit": Value Change {
        n156 = event-data() -> ()  [unwired: 1 in, 1 out]
        n157 = local read "HPSMO1"() -> (w383:refnum<class "Motion_Panel_State_Machine.lvclass">)
        n158 = Two Button Dialog(message="Exit Confirm") -> (T button?=w393:bool)  [unwired: 2 in]
        n159 = case shown="True" w393 {
          selector: w393 -> [w395 w422]
          tunnel: w392 -> [w399 w401]
          tunnel: w383 -> [_ w415]
          tunnel: w391 -> [w397 w420]
          tunnel: [w399 w411] -> w390
          tunnel: [w398 w421] -> w389
          tunnel: [w397 w420] -> w388
          tunnel: w387 -> [w398 w421]
          tunnel: w386 -> [w396 w419]
          tunnel: [w396 w419] -> w385
          tunnel: [w395 w422] -> w384
          tunnel: w382 -> [_ w403]
          frame False {
          }
          frame True {
            # "Remove Parent State with Last"
            n160 = call-dynamic "Get_Child_State.vi"("error in (no error)"=w401, "Hyper_State_Machine in"=w403) -> ("error out"=w408:errorcluster, "Child_State"=w406:refnum<class "State_Interface.lvclass">[], "Hyper_State_Machine out"=w407:refnum<class "Hyper_State_Machine.lvclass">)  [unwired: 5 in, 2 out]
            n161 = Build Array (concatenate)(w407, w406) -> (w409:refnum<class "State_Interface.lvclass">[])
            n162 = for {
              shift-right: [w429] -> w400
              shift-left: w408 -> [w424]
              tunnel: T3 {"Action_Mode (Get)"=enum."Set", "Action_Set (False)"=FALSE, "State_In (Wait)"="Lock"} ("Parameter") -> [w428]
              tunnel: refnum<class "Hyper_State_Machine.lvclass"> refnum ("HSMO1") -> [w427]
              tunnel: w409 -> [w423] mode=indexing
              n163 = To More Specific Class(target class=w427, reference=w423, error in=w424) -> (specific class reference=w426:refnum<class "Hyper_State_Machine.lvclass">, error out=w425:errorcluster)
              n164 = call-dynamic "State_Lock_Unlock.vi"("error in (no error)"=w425, "Parameter"=w428, "State_Machine_Class in"=w426) -> ("error out"=w429:errorcluster)  [unwired: 6 in, 2 out]
            }
            n165 = call-dynamic "Get_Child_Panel.vi"("error in (no error)"=w400, "Motion_Panel_State_Machine in"=w415) -> ("error out"=w418:errorcluster, "Child_Panel"=w412:refnum<class "Panel_Interface.lvclass">[], "Motion_Panel_State_Machine out"=w410:refnum<class "Motion_Panel_State_Machine.lvclass">)  [unwired: 5 in, 2 out]
            n166 = Build Array (concatenate)(w412, w410) -> (w417:refnum<class "Panel_Interface.lvclass">[])
            n167 = for {
              tunnel: w417 -> [w434] mode=indexing
              tunnel: refnum<class "Panel_Adaptive.lvclass"> refnum ("SSW_Panel_Adaptive.lvlibp:Panel_Adaptive.lvclass") -> [w432]
              shift-right: [w435] -> w402
              shift-left: w418 -> [w433]
              n168 = Preserve Run-Time Class(object in=w434, error in=w433, 2:w432) -> (object out=w431:refnum<class "Panel_Adaptive.lvclass">, error out=w430:errorcluster)
              n169 = call-dynamic "Panel_Destroy.vi"("error in (no error)"=w430, "Hyper_Panel_State_Machine in"=w431) -> ("error out"=w435:errorcluster)  [unwired: 9 in]
            }
            n170 = local read "Parent_State"() -> (w414:refnum<class "Hyper_State_Machine.lvclass">)
            n171 = call-dynamic "State_LIFO.vi"("error in (no error)"=w402, "State Machine"=T2 {"Command"="Exit", "Data"=variant}, "State_Machine_Class in"=w414) -> ("error out"=w411:errorcluster)  [unwired: 7 in, 1 out]
          }
        }
      }
    }
  }
  n172 = while {
    tunnel: [w458] -> w20
    tunnel: [w457] -> w18
    tunnel: w13 -> [w453]
    tunnel: w12 -> [w452]
    tunnel: [w446] -> w17
    tunnel: [w445] -> w16
    tunnel: w14 -> [w443]
    stop <- w436 stop-if-true
    # "Panel Object Handling Sample"
    n173 = local read "HSMO1"() -> (w467:refnum<class "Hyper_State_Machine.lvclass">)
    n174 = call-dynamic "Get_Current_State.vi"("error in (no error)"=w443, "Hyper_State_Machine in"=w467) -> ("error out"=w462:errorcluster, "Current_State"=w456:T2, "Hyper_State_Machine out"=w463:refnum<class "Hyper_State_Machine.lvclass">)  [unwired: 7 in]
    n175 = call-dynamic "State_Acquisition.vi"("error in (no error)"=w452, "State_Interval_Time(s)"="Main_Interval(s)", "Main_Machine_State_Class in"=w453) -> ("error out"=w441:errorcluster, "State"=w450:T2, "Main_Machine_State_Class out"=w442:refnum<class "Hyper_State_Machine.lvclass">)  [unwired: 2 in, 4 out]
    n176 = Unbundle By Name(w456) -> ("Command"=w454:string, "Data"=w455:variant)
    "Get_Current State_Sub Panel_1" <- w454
    n177 = Unbundle By Name(w450) -> ("Command"=w451:string, "Data"=w444:variant)
    "Current_Parent_State" <- w451
    n178 = call-dynamic "Get_State_ID.vi"("error in (no error)"=w462, "Hyper_State_Machine in"=w463) -> ("error out"=w465:errorcluster, "State_ID"=→"Sub Panel_1(HSMO_ID)":u32, "Hyper_State_Machine out"=w466:refnum<class "Hyper_State_Machine.lvclass">)  [unwired: 7 in]
    n179 = call <vilib>:"High Resolution Polling Wait.vi"("seconds to wait"="Main_Interval(s)") -> ()  [unwired: 10 in, 1 out]
    n180 = call-dynamic "Get_State_ID.vi"("error in (no error)"=w441, "Hyper_State_Machine in"=w442) -> ("error out"=w439:errorcluster, "State_ID"=→"Parent_State_ID":u32, "Hyper_State_Machine out"=w440:refnum<class "Hyper_State_Machine.lvclass">)  [unwired: 7 in]
    n181 = local read "Main_Active"() -> (w477:bool)
    n182 = case shown="\"Idle\", Default" w454 {
      tunnel: w465 -> [w540 w545 w583 w585]
      tunnel: w466 -> [w541 w546 w584 w586]
      tunnel: [w541 w546 w584 w586] -> w461
      tunnel: [w540 w545 w583 w585] -> w460
      tunnel: w455 -> [_ _ _ _]
      frame "Idle", Default {
      }
      frame "State_Interval" {
        n183 = local read "HPSMO3"() -> (w547:refnum<class "DIO_Panel_State_Machine.lvclass">)
        n184 = local read "HPSMO4-20"() -> (w544:refnum<class "Panel_Adaptive.lvclass">[])
        n185 = local read "HPSMO2"() -> (w548:refnum<class "Panel_Adaptive.lvclass">)
        n186 = local read "HPSMO1"() -> (w549:refnum<class "Motion_Panel_State_Machine.lvclass">)
        n187 = Array Size(array=w544) -> (size(s)=w543:i32)
        n188 = Decrement(x=w543) -> (x-1=w542:i32)
        n189 = Index Array(array=w544, index=w542) -> (element=w552:refnum<class "Panel_Adaptive.lvclass">)
        n190 = Build Array(w549, w548, w547) -> (w562:refnum<class "Panel_Adaptive.lvclass">[])
        n191 = for {
          tunnel: w562 -> [w582] mode=indexing
          tunnel: [w581] -> w561 mode=indexing
          n192 = call-dynamic "Panel_Get_All_Values.vi"("Hyper_Panel_State_Machine in"=w582) -> ("All_Values"=w581:variant[])  [unwired: 8 in, 2 out]
        }
        "All_Values" <- w561
        n193 = call-dynamic "Panel_Get_Values_Index.vi"("Control_Indexes(Tabbing Order)"=i32[] [3, 6], "Hyper_Panel_State_Machine in"=w548) -> ("error out"=w558:errorcluster, "Data_Values"=w559:variant[])  [unwired: 7 in, 1 out]
        n194 = call-dynamic "Panel_Get_Values_Index.vi"("Control_Indexes(Tabbing Order)"=i32[] [3, 6], "Hyper_Panel_State_Machine in"=w547) -> ("error out"=w580:errorcluster, "Data_Values"=w571:variant[])  [unwired: 7 in, 1 out]
        n195 = call-dynamic "Panel_Get_Values_Index.vi"("Control_Indexes(Tabbing Order)"=i32[] [3, 6] ("control indexes"), "Hyper_Panel_State_Machine in"=w549) -> ("error out"=w563:errorcluster, "Data_Values"=w570:variant[])  [unwired: 7 in, 1 out]
        n196 = call-dynamic "Panel_Get_Values_Index.vi"("Control_Indexes(Tabbing Order)"=i32[] [3, 6], "Hyper_Panel_State_Machine in"=w552) -> ("error out"=w553:errorcluster, "Data_Values"=w556:variant[])  [unwired: 7 in, 1 out]
        n197 = Index Array(array=w571) -> (element #1=w577:variant, element #2=w575:variant)  [unwired: 2 in]
        n198 = Index Array(array=w570) -> (element #1=w566:variant, element #2=w568:variant)  [unwired: 2 in]
        n199 = Index Array(array=w559) -> (element #1=w576:variant, element #2=w574:variant)  [unwired: 2 in]
        n200 = Index Array(array=w556) -> (element #1=w554:variant, element #2=w555:variant)  [unwired: 2 in]
        n201 = Variant To Data(error in=w563, Variant=w566) -> (data=→"Active 1":bool)  [unwired: 1 in, 1 out]
        n202 = Variant To Data(error in=w563, Variant=w568) -> (data=→"Timing 1":dbl)  [unwired: 1 in, 1 out]
        n203 = Variant To Data(error in=w558, Variant=w576) -> (data=→"Active 2":bool)  [unwired: 1 in, 1 out]
        n204 = Variant To Data(error in=w558, Variant=w574) -> (data=→"Timing 2":dbl)  [unwired: 1 in, 1 out]
        n205 = Variant To Data(error in=w580, Variant=w577) -> (data=→"Active 3":bool)  [unwired: 1 in, 1 out]
        n206 = Variant To Data(error in=w580, Variant=w575) -> (data=→"Timing 3":dbl)  [unwired: 1 in, 1 out]
        n207 = Variant To Data(error in=w553, Variant=w554) -> (data=→"Active 20":bool)  [unwired: 1 in, 1 out]
        n208 = Variant To Data(error in=w553, Variant=w555) -> (data=→"Timing 20":dbl)  [unwired: 1 in, 1 out]
      }
      frame "Error_Action" {
      }
      frame "Exit" {
      }
    }
    n209 = case shown="\"Idle\", Default" w451 {
      selector: w451 -> [_ _ _ _ w494 _ _ _ _ _]
      tunnel: w440 -> [w481 w484 w486 w490 w500 w506 w524 w526 w534 w538]
      tunnel: w439 -> [w482 w483 w485 w491 w497 w505 w523 w530 w533 w535]
      tunnel: w450 -> [_ _ _ _ _ _ _ _ _ _]
      tunnel: [w480 w484 w486 w490 w499 w504 w521 w526 w534 w537] -> w449
      tunnel: [w479 w483 w485 w488 w498 w507 w520 w527 w533 w536] -> w448
      tunnel: w444 -> [_ _ _ w492 _ _ _ w532 _ _]
      tunnel: "Main_Interval(s)" -> [_ _ _ _ w493 _ _ _ _ _]
      tunnel: [_ _ _ _ _ _ _ _ _ TRUE] -> w436
      frame "Idle", Default {
        n210 = call-dynamic "State_FIFO.vi"("error in (no error)"=w482, "State Machine[]"=T4 [{"Command"="Update_Child_Interval", "Data"=variant}], "State_Machine_Class in"=w481) -> ("error out"=w479:errorcluster, "State_Machine_Class out"=w480:refnum<class "Hyper_State_Machine.lvclass">)  [unwired: 7 in]
      }
      frame "State_Init" {
      }
      frame "State_Interval" {
      }
      frame "Block_Chain_Message" {
        n211 = Variant To Data(error in=w491, type="", Variant=w492) -> (data=→"Received State Message":string, error out=w488:errorcluster)
      }
      frame "Update_Child_Interval" {
        n212 = Bundle By Name(cluster=T5 {"Enable(True)"=TRUE, "Time Out_State Name"="", "Time Target (1s)"=0.0, "Time Out_Reply Message_State"="Child_State_Update"} ("Parameter"), "Time Out_State Name"=w494, "Time Target (1s)"=w493) -> (w495:T5)
        n213 = call-dynamic "State_Time_Out.vi"("error in (no error)"=w497, "Parameter"=w495, "State_Machine_Class in"=w500) -> ("error out"=w498:errorcluster, "State_Machine_Class out"=w499:refnum<class "Hyper_State_Machine.lvclass">)  [unwired: 5 in, 2 out]
      }
      frame "Child_State_Update" {
        n214 = call-dynamic "Get_Child_State.vi"("error in (no error)"=w505, "Hyper_State_Machine in"=w506) -> ("error out"=w502:errorcluster, "Child_State"=w503:refnum<class "State_Interface.lvclass">[], "Hyper_State_Machine out"=w504:refnum<class "Hyper_State_Machine.lvclass">, "Child_State#"=w501:u32)  [unwired: 5 in, 1 out]
        "Child_State#" <- w501
        n215 = for {
          shift-right: [w513] -> w510
          shift-left: w502 -> [w517]
          tunnel: w503 -> [w518] mode=indexing
          tunnel: refnum<class "Hyper_State_Machine.lvclass"> refnum ("HSMO1") -> [w516]
          tunnel: [w512] -> w511 mode=indexing
          n216 = Preserve Run-Time Class(object in=w518, error in=w517, 2:w516) -> (object out=w514:refnum<class "Hyper_State_Machine.lvclass">, error out=w515:errorcluster)
          n217 = call-dynamic "Get_State_ID.vi"("error in (no error)"=w515, "Hyper_State_Machine in"=w514) -> ("error out"=w513:errorcluster, "State_ID"=w512:u32)  [unwired: 7 in, 1 out]
        }
        "Child_State_ID" <- w511
        n218 = Decrement(x=w501) -> (x-1=w509:u32)
        n219 = property on="Panel_Index" class="DigNum (strict)"(error in=w510, "Maximum"=w509) -> (error out=w507:errorcluster)  [unwired: 1 in, 1 out]
      }
      frame "Lock" {
        n220 = call-dynamic "State_Lock_Unlock.vi"("error in (no error)"=w523, "Parameter"=T3 {"Action_Mode (Get)"=enum."Get", "Action_Set (False)"=FALSE, "State_In (Wait)"="Lock"}, "State_Machine_Class in"=w524) -> ("error out"=w520:errorcluster, "Action_Get"=→"Block_Chain_Lock":bool, "State_Machine_Class out"=w521:refnum<class "Hyper_State_Machine.lvclass">)  [unwired: 6 in]
      }
      frame "Dynamic_Release" {
        n221 = Variant To Data(error in=w530, type=refnum<class "Hyper_State_Machine.lvclass"> refnum ("State_Machine_Class in"), Variant=w532) -> (data=w529:refnum<class "Hyper_State_Machine.lvclass">, error out=w528:errorcluster)
        n222 = call-dynamic "State_Lock_Unlock.vi"("error in (no error)"=w528, "Parameter"=T3 {"Action_Mode (Get)"=enum."Set", "Action_Set (False)"=FALSE, "State_In (Wait)"="Wait"}, "State_Machine_Class in"=w529) -> ("error out"=w527:errorcluster)  [unwired: 6 in, 2 out]
      }
      frame "Error_Action" {
      }
      frame "Exit" {
        n223 = call-dynamic "State_Release.vi"("error in (no error)"=w535, "State_Machine_Class in"=w538) -> ("error out"=w536:errorcluster, "State_Machine_Class out"=w537:refnum<class "Hyper_State_Machine.lvclass">)  [unwired: 8 in]
      }
    }
    n224 = Not(x=w477) -> (.not. x?=→"Main_Active":bool)
    n225 = Get Date/Time In Seconds() -> (seconds since 1Jan1904=w475:timestamp)
    n226 = Get Date/Time String(seconds (now)=w475, want seconds? (F)=TRUE) -> (date string=w473:string, time string=w469:string)  [unwired: 1 in]
    n227 = Concatenate Strings("State Block Chain Framework ::  " ("string"), w473, " " ("string"), w469) -> (w471:string)
    n228 = control-ref of="This VI"() -> (w468:refnum<vi>)
    n229 = call-dynamic "Get_Running_Status.vi"("error in (no error)"=w460, "Hyper_State_Machine in"=w461) -> ("error out"=w457:errorcluster, "State_Running"=→"HSMO1 Running":bool, "Hyper_State_Machine out"=w458:refnum<class "Hyper_State_Machine.lvclass">)  [unwired: 7 in]
    n230 = call-dynamic "State_Error_Handling.vi"("error in (no error)"=w448, "Reply_State_Name"="Error_Action", "Handling_State(State_Acquisition)"=w450, "State_Machine_Class in"=w449) -> ("error out"=w446:errorcluster, "State_Machine_Class out"=w445:refnum<class "Hyper_State_Machine.lvclass">)  [unwired: 6 in]
    n231 = property class="VI"(reference=w468, "Front Panel.Title"=w471) -> ()  [unwired: 1 in, 2 out]
  }
  n232 = disable-structure shown="Enabled" {
    disable-tunnel: w18 -> [w589 w591]
    disable-tunnel: w20 -> [w588 _]
    disable-tunnel: [w587 w590] -> w19
    frame Disabled {
      n233 = call-dynamic "State_Destroy.vi"("error in (no error)"=w589, "State_Machine_Class in"=w588) -> ("error out"=w587:errorcluster)  [unwired: 9 in]
    }
    frame Enabled {
      n234 = call <vilib>:"Clear Errors.vi"("error in (no error)"=w591) -> ("error out"=w590:errorcluster)  [unwired: 5 in, 1 out]
    }
  }
  n235 = call-dynamic "State_Destroy.vi"("error in (no error)"=w17, "State_Machine_Class in"=w16) -> ("error out"=w15:errorcluster)  [unwired: 9 in]
  n236 = Merge Errors(w3, w4, w5, w6, w19, w15) -> (w2:errorcluster)
  n237 = call <vilib>:"Simple Error Handler.vi"("error in (no error)"=w2) -> ("error out"=w1:errorcluster)  [unwired: 4 in, 4 out]
  "error out" <- w1
  n238 = disable-structure shown="RUN_TIME_ENGINE==True" {
    disable-tunnel: w1 -> [_ _]
    frame condition #0 (active) {
    }
    frame condition #1 {
      n239 = Quit LabVIEW() -> ()  [unwired: 1 in]
    }
  }
